vi "FPGA Image Processing (Host).vi"() -> ()   [LabVIEW 2013]
uses:
  <vilib>/rvi/interface/nirviMethod/nirviMethod.xnode
  <vilib>/rvi/interface/nirviCloseFPGA/nirviCloseFPGA.xnode
  <vilib>/FPGAPlugInAG/Dynamic/niLvFpga_Close_Dynamic.vi
  <vilib>/FPGAPlugInAG/Dynamic/niLvFpga_Reset_Dynamic.vi
  <vilib>/FPGAPlugInAG/Dynamic/niLvFpga_Run_Dynamic.vi
  <vilib>/rvi/interface/nirviReadWriteControl/nirviReadWriteControl.xnode
  <vilib>/rvi/interface/Simulation/niFpgaSimulationCallBeginRW.vi
  <vilib>/rvi/errors/niLvFpgaAdjustHostInterfaceError.vi
  <vilib>/userdefined/High Color/nirio_resource_hc.ctl
panel:
  in  "stop":bool
  in  "Bitfile path":path
  in  "RIO Device":T1="RIO0"
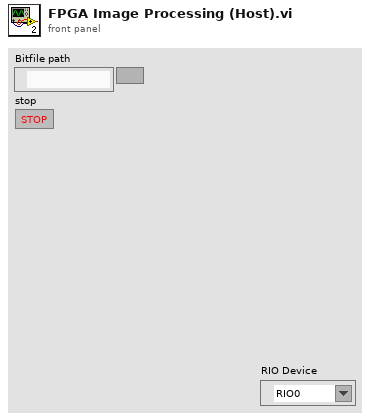
[diagram p1: front panel]
types:
  T1 = typedef "nirio_resource_hc.ctl" = tag
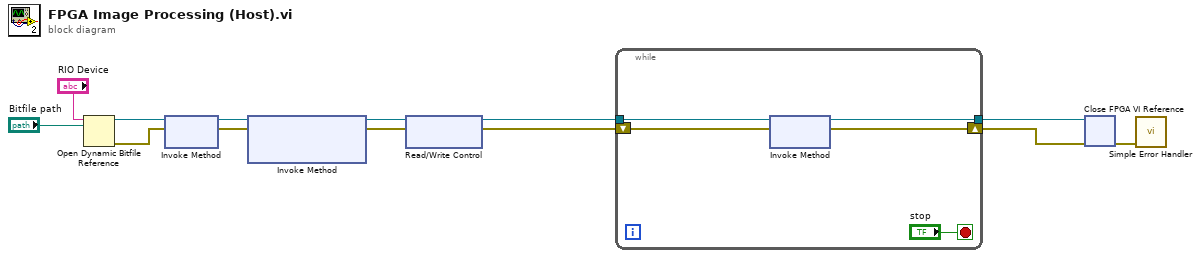
[diagram p0: block diagram]
diagram:
  n1 = Open Dynamic Bitfile Reference(0:"RIO Device", 1:"Bitfile path") -> (5:w8:refnum<k20>, 8:w7:errorcluster)  [unwired: 3 in]
  n2 = xnode "Invoke Method"("FPGA VI Reference In"=w8, "error in"=w7) -> ("FPGA VI Reference Out"=w6:refnum<k20>, "error out"=w5:errorcluster)
  n3 = xnode "Invoke Method"("FPGA VI Reference In"=w6, "error in"=w5) -> ("FPGA VI Reference Out"=w4:refnum<k20>, "error out"=w2:errorcluster)  [unwired: 1 in]
  n4 = xnode "Read/Write Control"("FPGA VI Reference In"=w4, "error in"=w2) -> ("FPGA VI Reference Out"=w3:refnum<k20>, "error out"=w1:errorcluster)  [unwired: 1 out]
  n5 = while {
    tunnel: w3 -> [w18]
    tunnel: [w16] -> w11
    shift-right: [w15] -> w10
    shift-left: w1 -> [w17]
    stop <- "stop" stop-if-true
    n6 = xnode "Invoke Method"("FPGA VI Reference In"=w18, "error in"=w17) -> ("FPGA VI Reference Out"=w16:refnum<k20>, "error out"=w15:errorcluster)
  }
  n7 = xnode "Close FPGA VI Reference"("FPGA VI Reference In"=w11, "error in"=w10) -> ("error out"=w9:errorcluster)
  n8 = call <vilib>:"Simple Error Handler.vi"("error in (no error)"=w9) -> ()  [unwired: 4 in, 5 out]
